vi "Monitors_v00.vi"(8 "wfm":waveform(dbl)[](array[waveform]), 9 "Shot noise start":bool, 10 "Monitor Switches":T1, 11 "IIR filter specifications":T2={"Topology"=enum."Butterworth", "Type"=enum."Lowpass", "Order"=1, "Lower Fc"=100.0, "Upper Fc"=200.0, "PB Ripple"=1.0, "SB Attenuation"=60.0} {"PB Ripple" format="%0.2f"; "SB Attenuation" format="%0.2f"; "Lower Fc" format="%0.2p"; "Upper Fc" format="%0.2p"}) -> (0 "covariance":dbl, 1 "conditional variance":dbl, 2 "Variance 2 normalised to SNL":dbl(graph), 3 "Variance 1 normalised to SNL":dbl(graph), 4 "Signal 1":dbl[](graph), 6 "Signal 2":dbl[](graph))   [LabVIEW 2013]
uses:
  Strict Type Defs/Monitor switches.ctl
  <vilib>/Analysis/5stat.llb/RMS (DBL).vi
  <vilib>/Analysis/baseanly.llb/Mean (DBL).vi
  <vilib>/measure/macond.llb/IIR Filter for N Chan.vi
  Global VIs/shotnoise.vi
  <vilib>/measure/NI_MAPro.lvlib
  <vilib>/Analysis/NI_AALPro.lvlib
  <vilib>/Analysis/NI_AALBase.lvlib
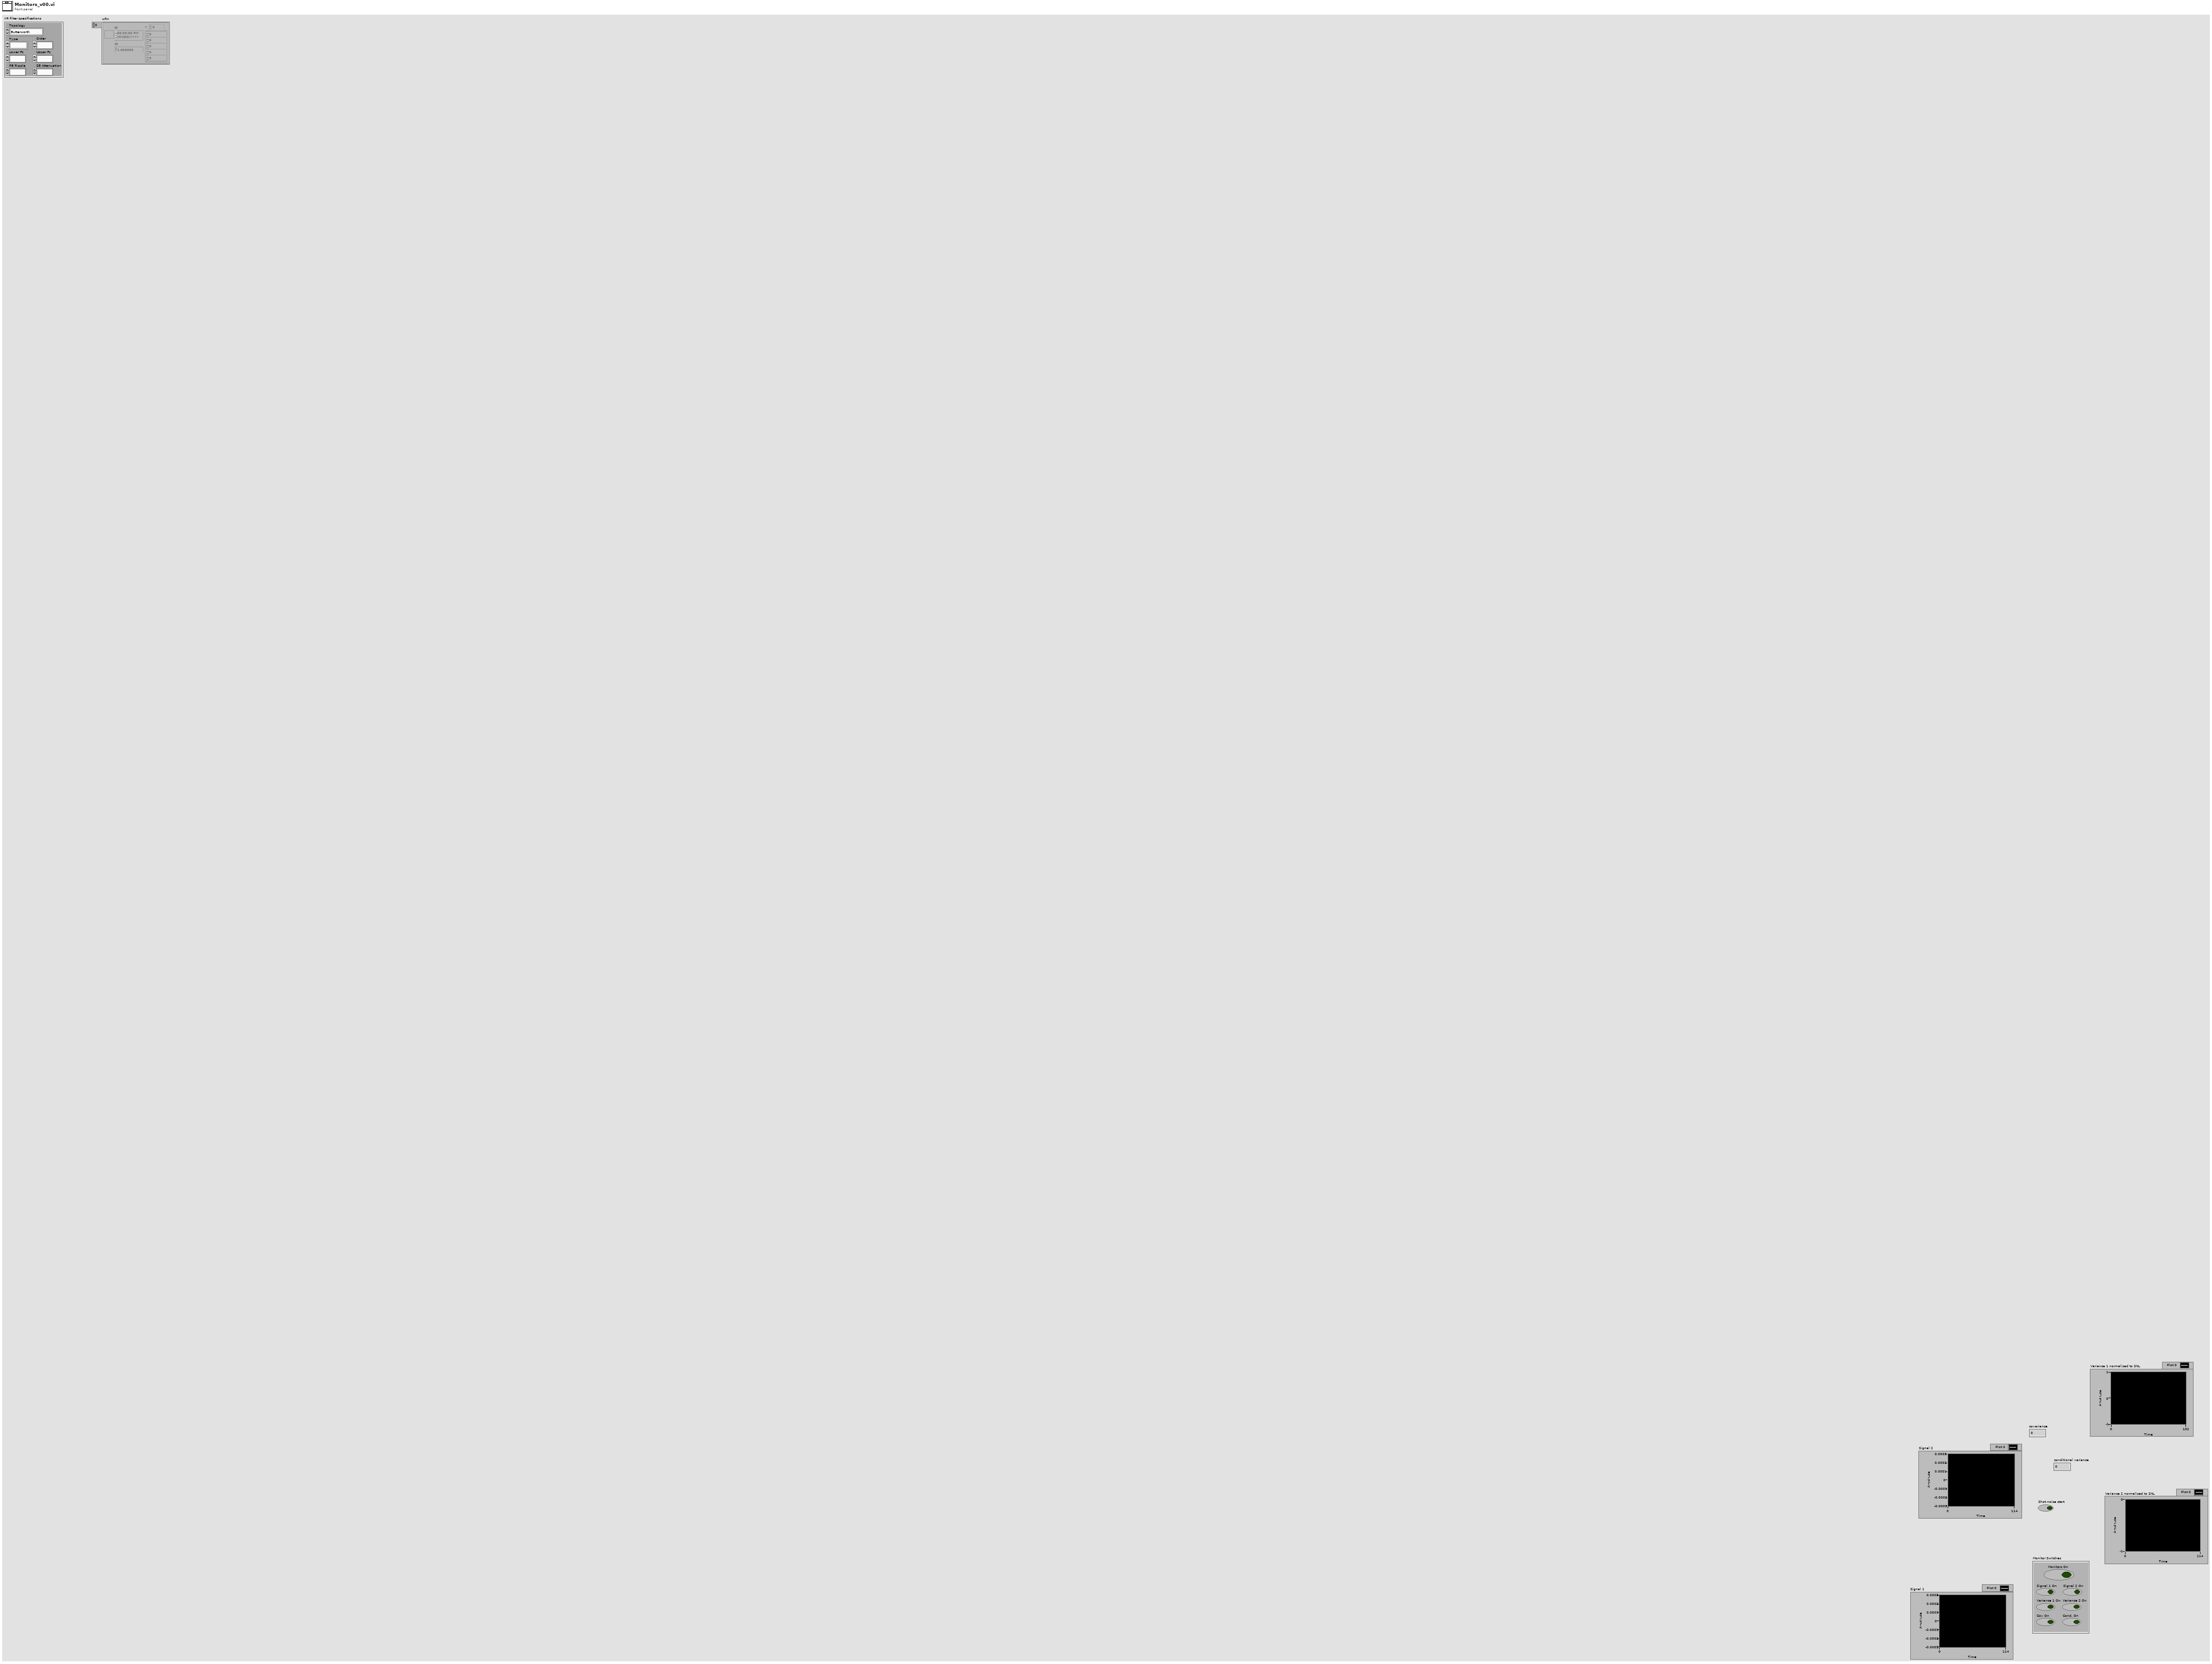
[diagram p1: front panel]
types:
  T1 = typedef "Monitor switches.ctl" = cluster{"Signal 1 On":bool, "Signal 2 On":bool, "Variance 1 On":bool, "Variance 2 On":bool, "Cov On":bool, "Cond. On":bool, "Monitors On":bool}
  T2 = cluster{"Topology":enum16{"Off", "Butterworth", "Chebyshev", "Inverse Chebyshev", "Elliptic", "Bessel"}, "Type":enum16{"Lowpass", "Highpass", "Bandpass", "Bandstop"}, "Order":i32, "Lower Fc":dbl, "Upper Fc":dbl, "PB Ripple":dbl, "SB Attenuation":dbl}
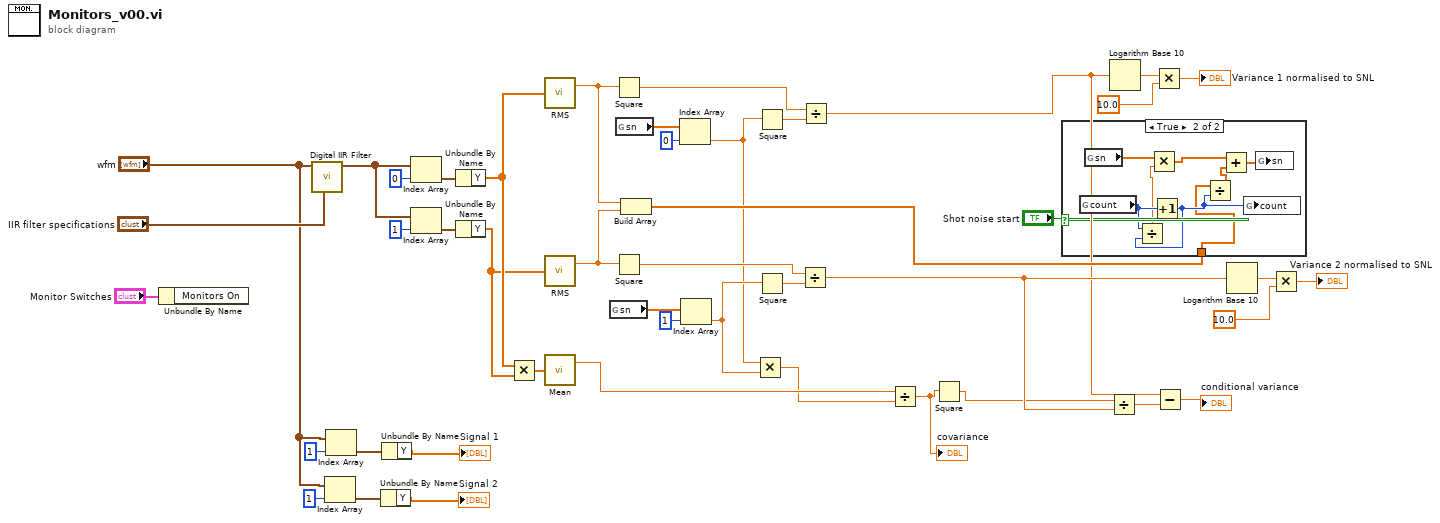
[diagram p0: block diagram]
diagram:
  n1 = Unbundle By Name("Monitor Switches") -> ()  [unwired: 1 out]
  n2 = call-poly <vilib>:"Digital IIR Filter.vi"("IIR filter specifications"="IIR filter specifications", "signal(s) in"="wfm") -> ("signal(s) out"=w7:waveform(dbl)[])  [unwired: 4 in, 5 out]
  n3 = Index Array(array="wfm", index=1) -> (element=w5:waveform(dbl))
  n4 = Index Array(array="wfm", index=1) -> (element=w2:waveform(dbl))
  n5 = Unbundle By Name(w5) -> ("Y"=→"Signal 2":dbl[])
  n6 = Unbundle By Name(w2) -> ("Y"=→"Signal 1":dbl[])
  n7 = Index Array(array=w7, index=0) -> (element=w16:waveform(dbl))
  n8 = Index Array(array=w7, index=1) -> (element=w21:waveform(dbl))
  n9 = Unbundle By Name(w16) -> ("Y"=w41:dbl[])
  n10 = Unbundle By Name(w21) -> ("Y"=w36:dbl[])
  n11 = Multiply(x=w41, y=w36) -> (x*y=w39:dbl[])
  n12 = call-poly <vilib>:"RMS.vi"("X"=w41) -> ("rms value"=w34:dbl)  [unwired: 1 out]
  n13 = call-poly <vilib>:"RMS.vi"("X"=w36) -> ("rms value"=w37:dbl)  [unwired: 1 out]
  n14 = call-poly <vilib>:"Mean.vi"("X"=w39) -> ("mean"=w40:dbl)  [unwired: 1 out]
  n15 = global read "shotnoise.vi" "sn"() -> (w19:dbl[])
  n16 = Square(x=w34) -> (x^2=w35:dbl)
  n17 = Square(x=w37) -> (x^2=w38:dbl)
  n18 = global read "shotnoise.vi" "sn"() -> (w18:dbl[])
  n19 = Build Array(w34, w37) -> (w33:dbl[])
  n20 = Index Array(array=w18, index=0) -> (element=w29:dbl)
  n21 = Index Array(array=w19, index=1) -> (element=w30:dbl)
  n22 = Multiply(x=w29, y=w30) -> (x*y=w31:dbl)
  n23 = Square(x=w29) -> (x^2=w26:dbl)
  n24 = Square(x=w30) -> (x^2=w28:dbl)
  n25 = Divide(x=w38, y=w28) -> (x/y=w32:dbl)
  n26 = Divide(x=w35, y=w26) -> (x/y=w27:dbl)
  n27 = Divide(x=w40, y=w31) -> (x/y=w42:dbl)
  "covariance" <- w42
  n28 = Square(x=w42) -> (x^2=w23:dbl)
  n29 = case shown="True" "Shot noise start" {
    tunnel: w33 -> [_ w47]
    frame False {
    }
    frame True {
      n30 = global read "shotnoise.vi" "count"() -> (w52:i64)
      n31 = global read "shotnoise.vi" "sn"() -> (w51:dbl[])
      n32 = Increment(x=w52) -> (x+1=w48:i64)
      n33 = Divide(x=w52, y=w48) -> (x/y=w50:dbl)
      n34 = Multiply(x=w51, y=w50) -> (x*y=w49:dbl[])
      n35 = Divide(x=w47, y=w48) -> (x/y=w46:dbl[])
      n36 = Add(x=w49, y=w46) -> (x+y=w53:dbl[])
      n37 = global write "shotnoise.vi" "count"(w48) -> ()
      n38 = global write "shotnoise.vi" "sn"(w53) -> ()
    }
  }
  n39 = Divide(x=w23, y=w32) -> (x/y=w24:dbl)
  n40 = Logarithm Base 10(1:w27) -> (0:w8:dbl)
  n41 = Multiply(x=w8, y=10.0) -> (x*y=→"Variance 1 normalised to SNL":dbl)
  n42 = Subtract(x=w27, y=w24) -> (x-y=→"conditional variance":dbl)
  n43 = Logarithm Base 10(1:w32) -> (0:w11:dbl)
  n44 = Multiply(x=w11, y=10.0) -> (x*y=→"Variance 2 normalised to SNL":dbl)
